vi "Read Logger Stop Msg.vi"(8 "error in (no error)":errorcluster, 11 "Logger in":refnum<class "Generic Logger.lvclass">) -> (0 "error out":errorcluster, 2 "Logger Stop Msg":refnum<queue>, 3 "Logger out":refnum<class "Generic Logger.lvclass">)   [LabVIEW 2020, in "Logging.lvlib" / "Generic Logger.lvclass"]
uses:
  Generic Logger.lvclass
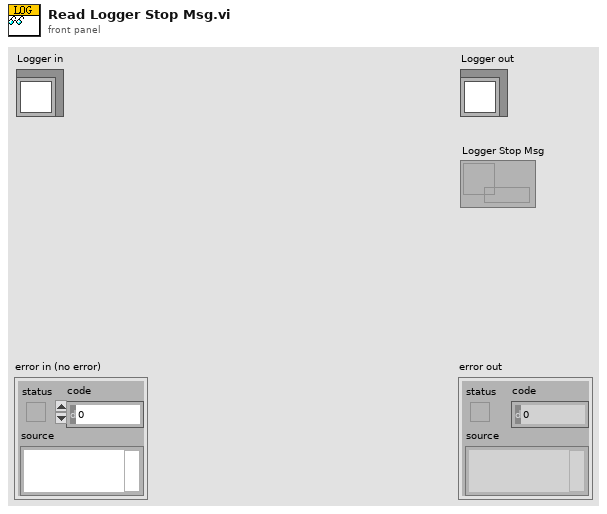
[diagram p1: front panel]
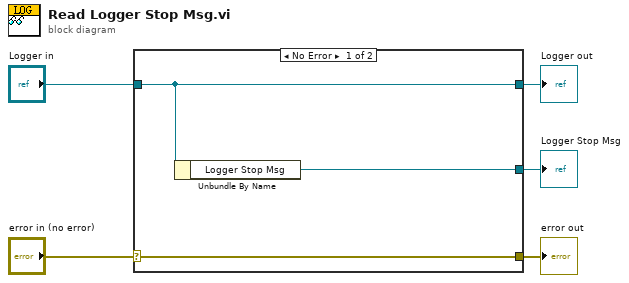
[diagram p0: block diagram]
diagram:
  n1 = case shown="No Error" "error in (no error)" {
    selector: "error in (no error)" -> [w8 w9]
    tunnel: [w8 w9] -> w4
    tunnel: [w7 w10] -> w2
    tunnel: "Logger in" -> [w7 w10]
    tunnel: [w6 _] -> w1
    frame No Error {
      n2 = Unbundle By Name(w7) -> ("Logger Stop Msg"=w6:refnum<queue>)
    }
    frame Error {
    }
  }
  "error out" <- w4
  "Logger out" <- w2
  "Logger Stop Msg" <- w1
